vi "updateCheckSum.vi"(8 "error in (no error)":errorcluster, 10 "message":string=".0101WatchDog", 11 "CoolerSerialCommand in":refnum<class "CoolerSerialCommand.lvclass">) -> (0 "error out":errorcluster, 2 "result message":string, 3 "CoolerSerialCommand out":refnum<class "CoolerSerialCommand.lvclass">)   [LabVIEW 2016, in "CoolerSerialCommand.lvclass"]
uses:
  CoolerSerialCommand.lvclass
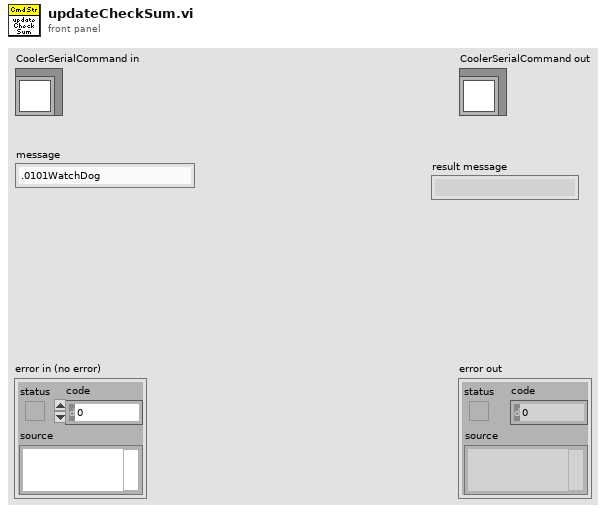
[diagram p1: front panel]
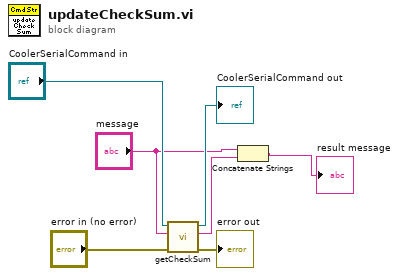
[diagram p0: block diagram]
diagram:
  n1 = call "getCheckSum.vi"("error in (no error)"="error in (no error)", "response"="message", "CoolerSerialCommand in"="CoolerSerialCommand in") -> ("error out"=→"error out":errorcluster, "Checksum"=w1:string, "CoolerSerialCommand out"=→"CoolerSerialCommand out":refnum<class "CoolerSerialCommand.lvclass">)  [unwired: 6 in]
  n2 = Concatenate Strings("message", w1) -> (→"result message":string)
